vi "PathSup2Hatches.vi"(11 "PathSupOut":T2) -> (3 "Hatches":T1(array[cluster]))   [LabVIEW 2014]
uses:
  TypeDefs/PathSupreme.ctl
  PSup2SCAN/Sub/VelocityProfile.ctl
  PSup2SCAN/Sub/PathCut.ctl
  PSup2SCAN/Sub/Segment.ctl
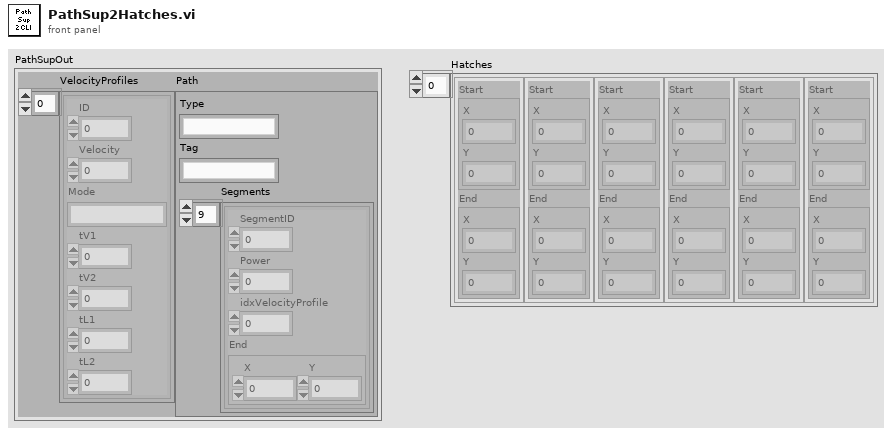
[diagram p1: front panel]
types:
  T1 = cluster{"Start":cluster{"X":dbl, "Y":dbl}, "End":cluster{"X":dbl, "Y":dbl}}[]
  T2 = typedef "PathSupreme.ctl" = cluster{"VelocityProfiles":T3[], "Path":T4}
  T3 = typedef "VelocityProfile.ctl" = cluster{"ID":u32, "Velocity":dbl, "Mode":string, "tV1":u32, "tV2":u32, "tL1":u32, "tL2":u32}
  T4 = typedef "PathCut.ctl" = cluster{"Type":string, "Tag":string, "Segments":T5[]}
  T5 = typedef "Segment.ctl" = cluster{"SegmentID":u16, "Power":sgl, "idxVelocityProfile":u16, "End":cluster{"X":sgl, "Y":sgl}}
  T6 = cluster{"Start":cluster{"X":dbl, "Y":dbl}, "End":cluster{"X":dbl, "Y":dbl}}
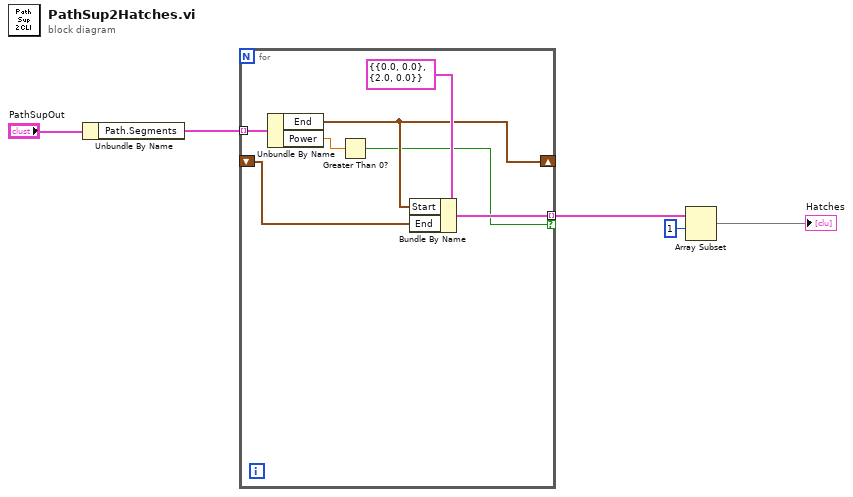
[diagram p0: block diagram]
diagram:
  n1 = Unbundle By Name("PathSupOut") -> ("Path.Segments"=w4:T5[])
  n2 = for {
    tunnel: w4 -> [w11] mode=indexing
    shift-right: [w9] -> _
    shift-left: _ -> [w6]
    tunnel: [w8] -> w3 mode=indexing if=w7
    n3 = Unbundle By Name(w11) -> ("End"=w9:cluster{"X":sgl, "Y":sgl}, "Power"=w12:sgl)
    n4 = Greater Than 0?(x=w12) -> (x > 0?=w7:bool)
    n5 = Bundle By Name(cluster=T6 {"Start"={"X"=0.0, "Y"=0.0}, "End"={"X"=2.0, "Y"=0.0}} ("Line"), "Start"=w9, "End"=w6) -> (w8:T6)
  }
  n6 = Array Subset(array=w3, index=1) -> (→"Hatches":T1)  [unwired: 1 in]
